vi "DAS.vi"() -> ()   [LabVIEW 2012]
uses:
  <vilib>/Utility/error.llb/DialogType.ctl
  SITK/Documents/SIToolkit/LabVIEW/Examples2012_4_1_0_4/Open-Close/CamHandle.vi
panel:
  in  "Record 3":bool
  in  "bUseBuffer1 3":bool
  in  "bUseBuffer0 3":bool
  in  "Record 2":bool
  in  "bUseBuffer1 2":bool
  in  "bUseBuffer0 2":bool
  in  "bUseBuffer0":bool
  in  "bUseBuffer1":bool
  in  "Open StructureIn":T1={"Size"=88, "InterfaceType"=0, "Camera Number"=0, "CameraNumAtInterface"=0, "OpenFlags"=[], "OpenDWFlags"=[], "OpenPtrs"=[]}
  out "Bits/pixel":u16
  out "BufNr1":i16
  out "BufNr0":i16
  in  "error in (no error)":errorcluster
  in  "Camera Handle 2":u32
  in  "File and Display Name 2":string
  in  "error in (no error) 2":errorcluster
  in  "Errors":errorcluster
  in  "?":T2(tab)
  out "Database Output":string
  out "Elapsed Time":u32
  in  "Image Tabs":T3(tab)
  out "Normalized Image":dbl[][](graph)
  out "Atoms":i16[][](graph)
  out "No Atoms":i16[][](graph)
  out "Dark Field":i16[][](graph)
  in  "?":T4(tab)
  in  "Cycle Devices (Red)\nAcquisition (Blue)":bool
  in  "?":bool
  in  "Scaling":dbl(slide)=0.0016108638057548662 scale=0.001..0.1
  in  "PF Scale":dbl(slide)=0.002000674655718671 scale=0.001..10.0
  in  "ADC Gain":i32=-1 min=-1 step=1
  in  "ADC Speed":i32=-1 min=-3 step=1
  in  "Exposure (sec)":dbl format="%.3f"
  in  "Number of Images":u32=1
  in  "Number of Accumulations":u32=1
  in  "Acquire / Focus Flag":u32(ring)=2 items=["Synchronous Focus Mode"=1, "Synchronous NFrame Mode"=2, "Asynchronous Mode"=3, "Sequence Mode"=4]
  in  "Timing Mode":u32(ring)=4 items=["Free Run"=1, "Trigger First"=2, "Strobe"=3, "Bulb"=4, "Variable"=5, "Flash"=6]
  in  "Trigger Edge":u32(ring)=1 items=["Rising"=1, "Falling"=2]
  in  "Milliseconds Between Shots":u32=200
  in  "InterfaceType":u16(ring)=6 items=["IEEE1394 - Firewire", "IEEE1394/Firewire", "Matrox Helios Camera Link", "Silicon Software ME3 Camera Link", "National Instruments Camera Link", "Gigabit Ethernet", "USB", "Reserved", "Reserved", "Reserved", "Generic Camera Link with CLSER.DLL"]
  in  "Rate":i32
  in  "ROIX1":u16=1 min=1
  in  "ROIY1":u16=1 min=1
  in  "ROIY0":u16=1 min=1
  in  "ROIX0":u16=1 min=1
  in  "DelayTimeBase":u16(ring)=2 items=["nanoseconds", "microseconds", "milliseconds"]
  in  "ExposureTimeBase":u16(ring)=1 items=["nanoseconds", "microseconds", "milliseconds"]
  in  "Exposure":u32=30
  in  "Delay":u32=100
  in  "StorageMode":bool
  in  "TriggerMode":u16(ring)=2 items=["Auto", "Software", "External sequence start ", "External exposure control"]
  out "Top of Chamber Monitor":dynamicdata(graph)
  in  "Image Tabs 2":T3(tab)
  out "Intensity Graph":dbl[][](graph)
  out "PF Atoms":u16[][](graph)
  out "PF No Atoms":u16[][](graph)
  out "PF Dark":u16[][](graph)
  # "Data Acquisition Suite v 1.3"
  # "Basic Output"
  # "Image Viewer"
  # "Image Viewer"
  # "DAS Mode Select"
  # "Stop Button"
  # "Experiment Setup"
  # "Advanced Setup"
  # "For everyday use, Number of Accumulations should be 1"
  # "Triggering Setup"
  # "Basic Setup for PixelFly"
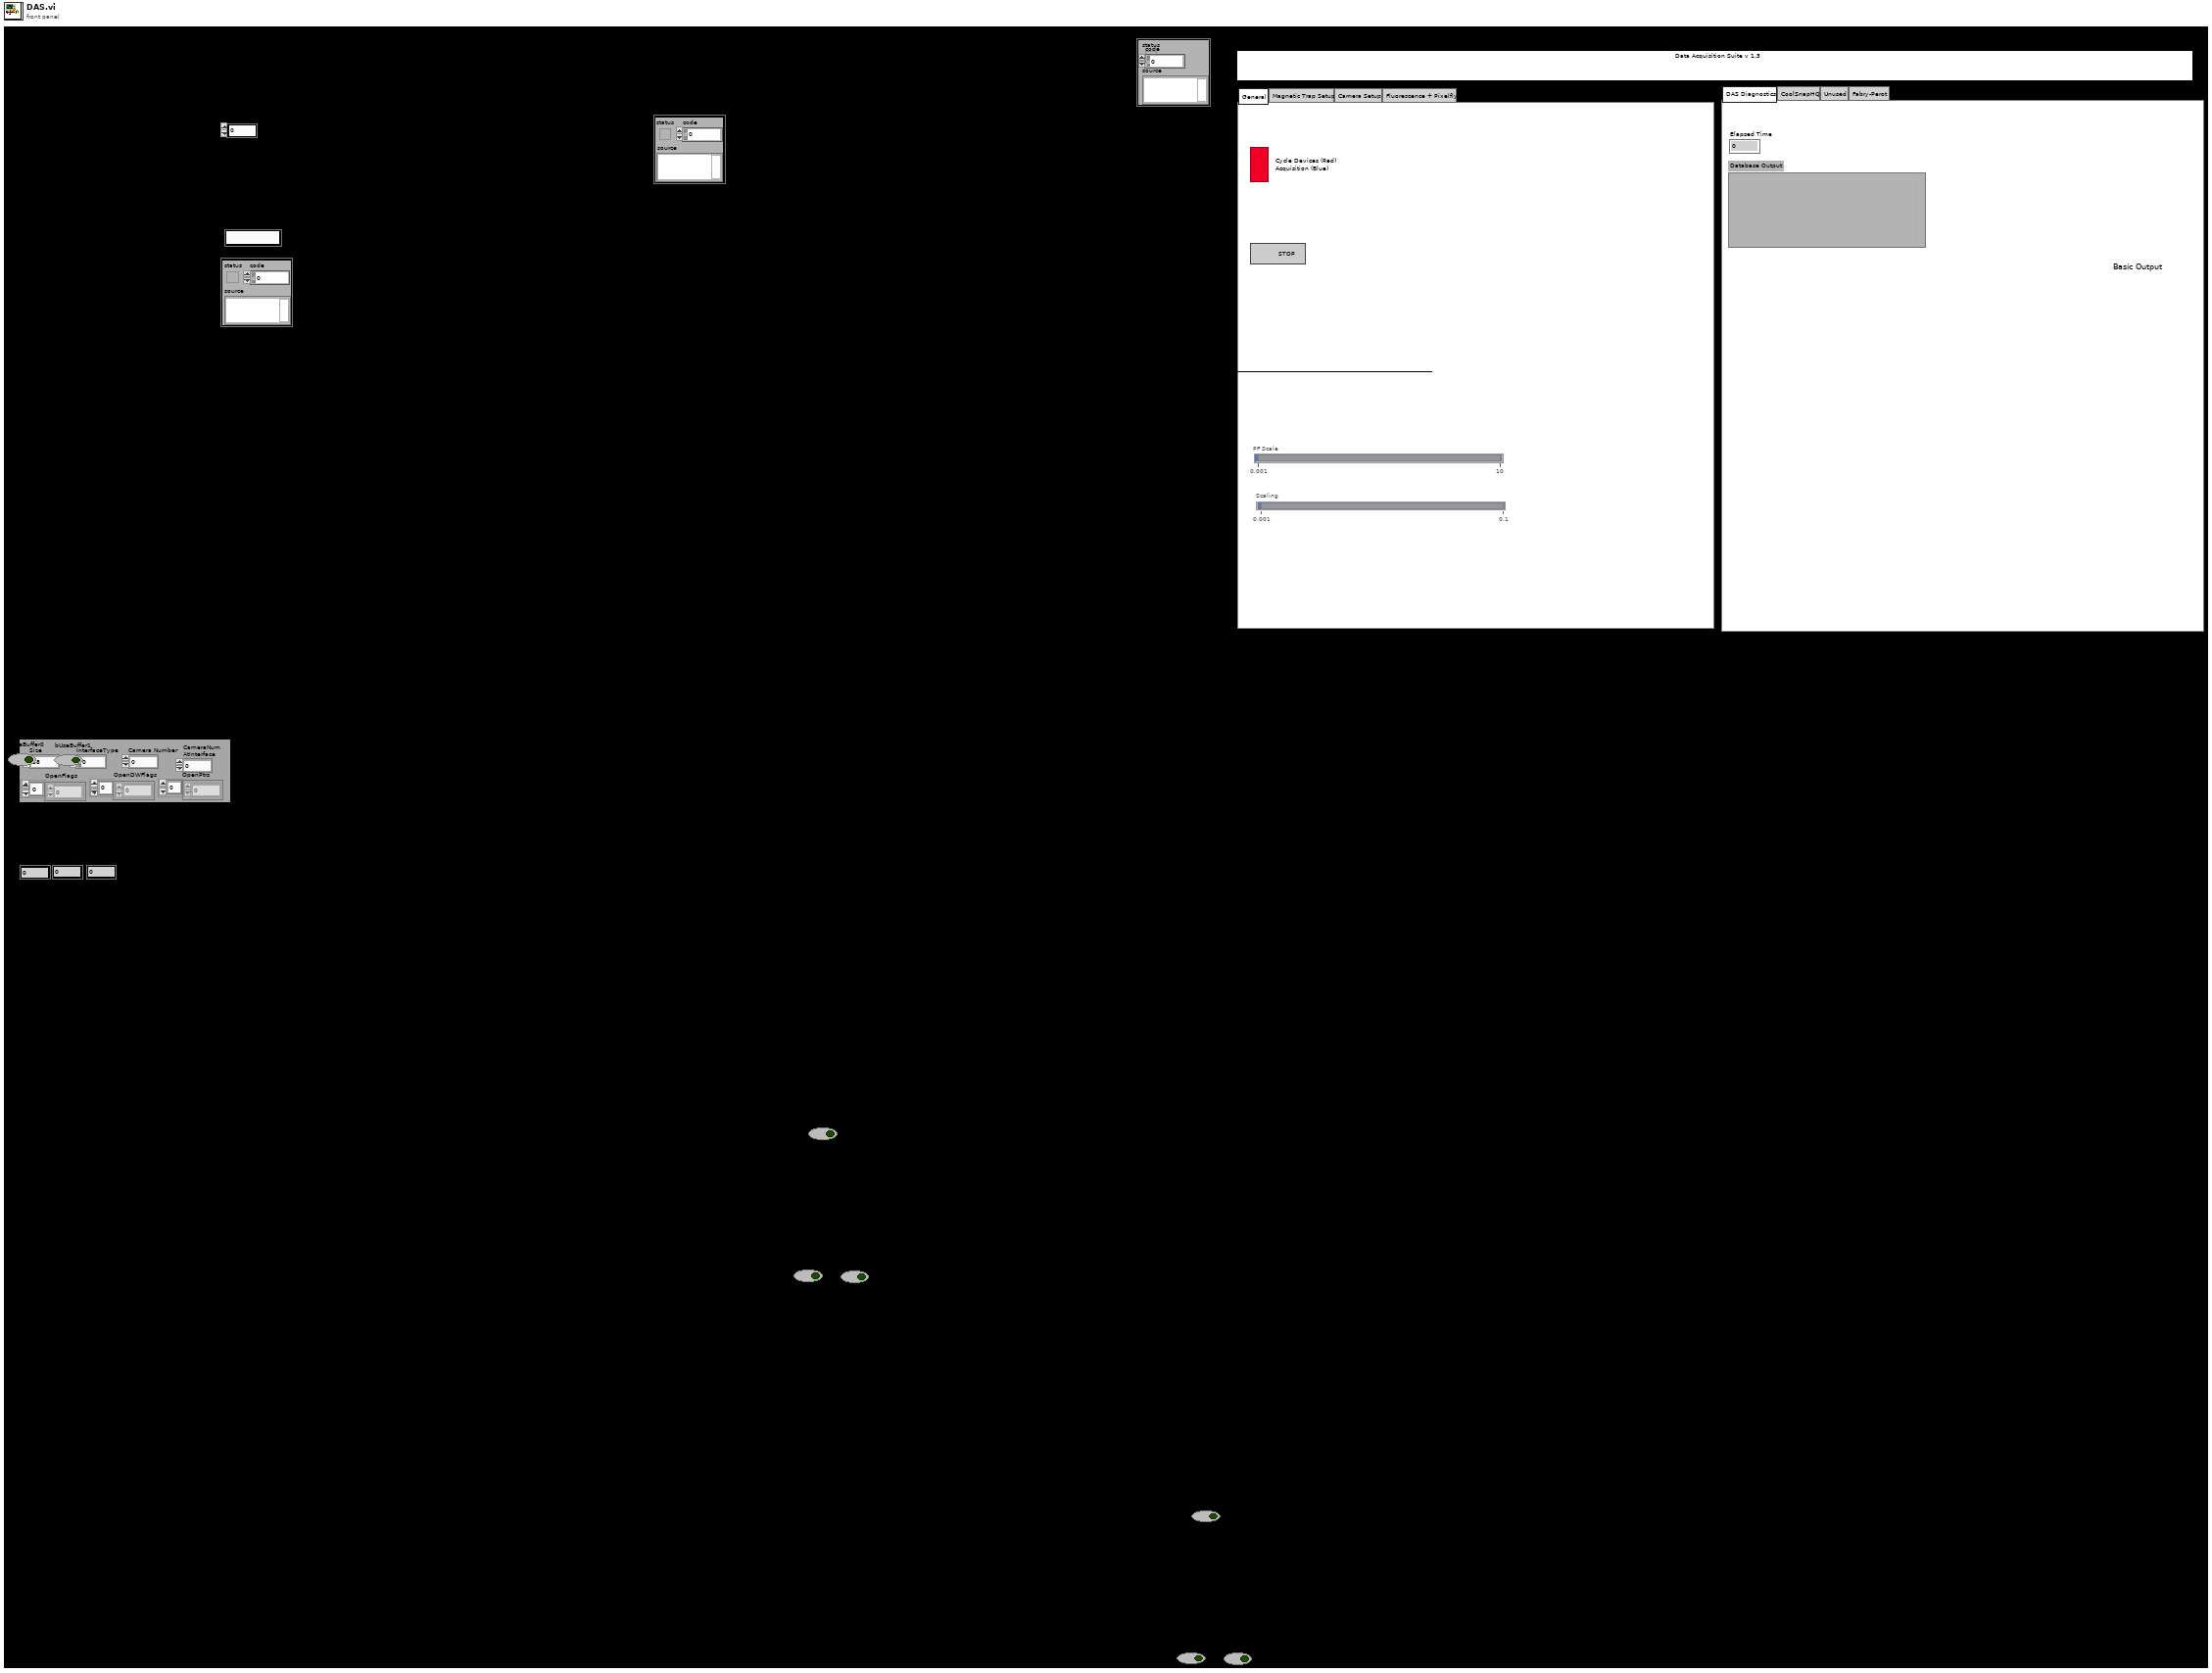
[diagram p1: front panel]
types:
  T1 = cluster{"Size":u16, "InterfaceType":u16, "Camera Number":u16, "CameraNumAtInterface":u16, "OpenFlags":u16[], "OpenDWFlags":u32[], "OpenPtrs":u32[]}
  T2 = enum32{"DAS Diagnostics", "CoolSnapHQ", "Unused", "Fabry-Perot"}
  T3 = enum32{"Composite Image", "Atoms", "No Atoms", "Dark Field"}
  T4 = enum32{"General", "Magnetic Trap Setup", "Camera Setup", "Fluorescence + Pixelfly"}
  T5 = enum16{"open", "replace", "create", "open or create", "replace or create", "replace or create with confirmation"}
  T6 = enum16{"big-endian, network order", "native, host order", "little-endian"}
  T7 = typedef "DialogType.ctl" = u16
  T8 = cluster{"Size":u16, "CamType":u16, "CamSubType":u16, "SerialNumber":u32, "HWVersion":u32, "FWVersion":u32, "InterfaceType":u16, "HardwareVersion":cluster{"BoardNum":u16, "HWVersions":cluster{"BoardName":string, "BatchNumber":u16, "MinorRevision":u8, "MajorRevision":u8, "Variant":u16}[]}, "FirmwareVersion":cluster{"DeviceNum":u16, "FWVersions":cluster{"DeviceName":string, "MinorRevision":u8, "MajorRevision":u8, "Variant":u16}[]}}
  T9 = cluster{"Size":u16, "SensorTypeDESC":u16, "SensorSubtypeDESC":u16, "MaxHorizontalResStdDESC":u16, "MaxVerticalResStdDESC":u16, "MaxHorizontalResExtDESC":u16, "MaxVerticalResExtDESC":u16, "DynResDESC":u16, "MaxBinHorzDESC":u16, "BinHorzStepDESC":bool, "MaxBinVertDESC":u16, "BinVertStepDESC":bool, "ROIHorzStepDESC":u16, "ROIVertStepDESC":u16, "NumADCDESC":u16, "IRDESC":bool, "MinDelayDESC":u32, "MaxDelayDESC":u32, "MinDelayStepDESC":u32, "MinExpoDESC":u32, "MaxExpoDESC":u32, "MinExpoStepDESC":u32, "MinDelayIRDESC":u32, "MaxDelayIRDESC":u32, "MinExpoIRDESC":u32, "MaxExpoIRDESC":u32, "TimeTableDESC":bool, "DoubleImageDESC":bool, "MinCoolSetDESC":i16, "MaxCoolSetDESC":i16, "MDefaultCoolSetDESC":i16, "PowerDownModeDESC":bool, "OffsetRegDESC":bool, "ColorPattern":cluster{"UpperLeftColor":u8, "UpperRightColor":u8, "LowerLeftColor":u8, "LowerRightColor":u8}, "PatternTypeDESC":bool, "PixelRates":u32[], "CoversionFactors":u16[], "Reserved":u32[], "NoiseFilterCapable":bool, "HotPixelCapable":bool, "HotPixelWithNoiseFilter":bool, "ASCIITimeCapable":bool, "Extended Description":bool, "Get Extended":bool, "Reserved Flag 1":bool, "Reserved Flag 2":bool}
  T10 = cluster{"Camera Handle":u32, "File Handle":u32, "Display Handle":u32, "Image Handle":u32}
  T11 = cluster{u16[][], "XResAct":u16, "YResAct":u16, "BufNrOut":i16, "BufNrOut":i16, "ErrorOut":errorcluster, "hout":u64, "Bits/pixel":u16}
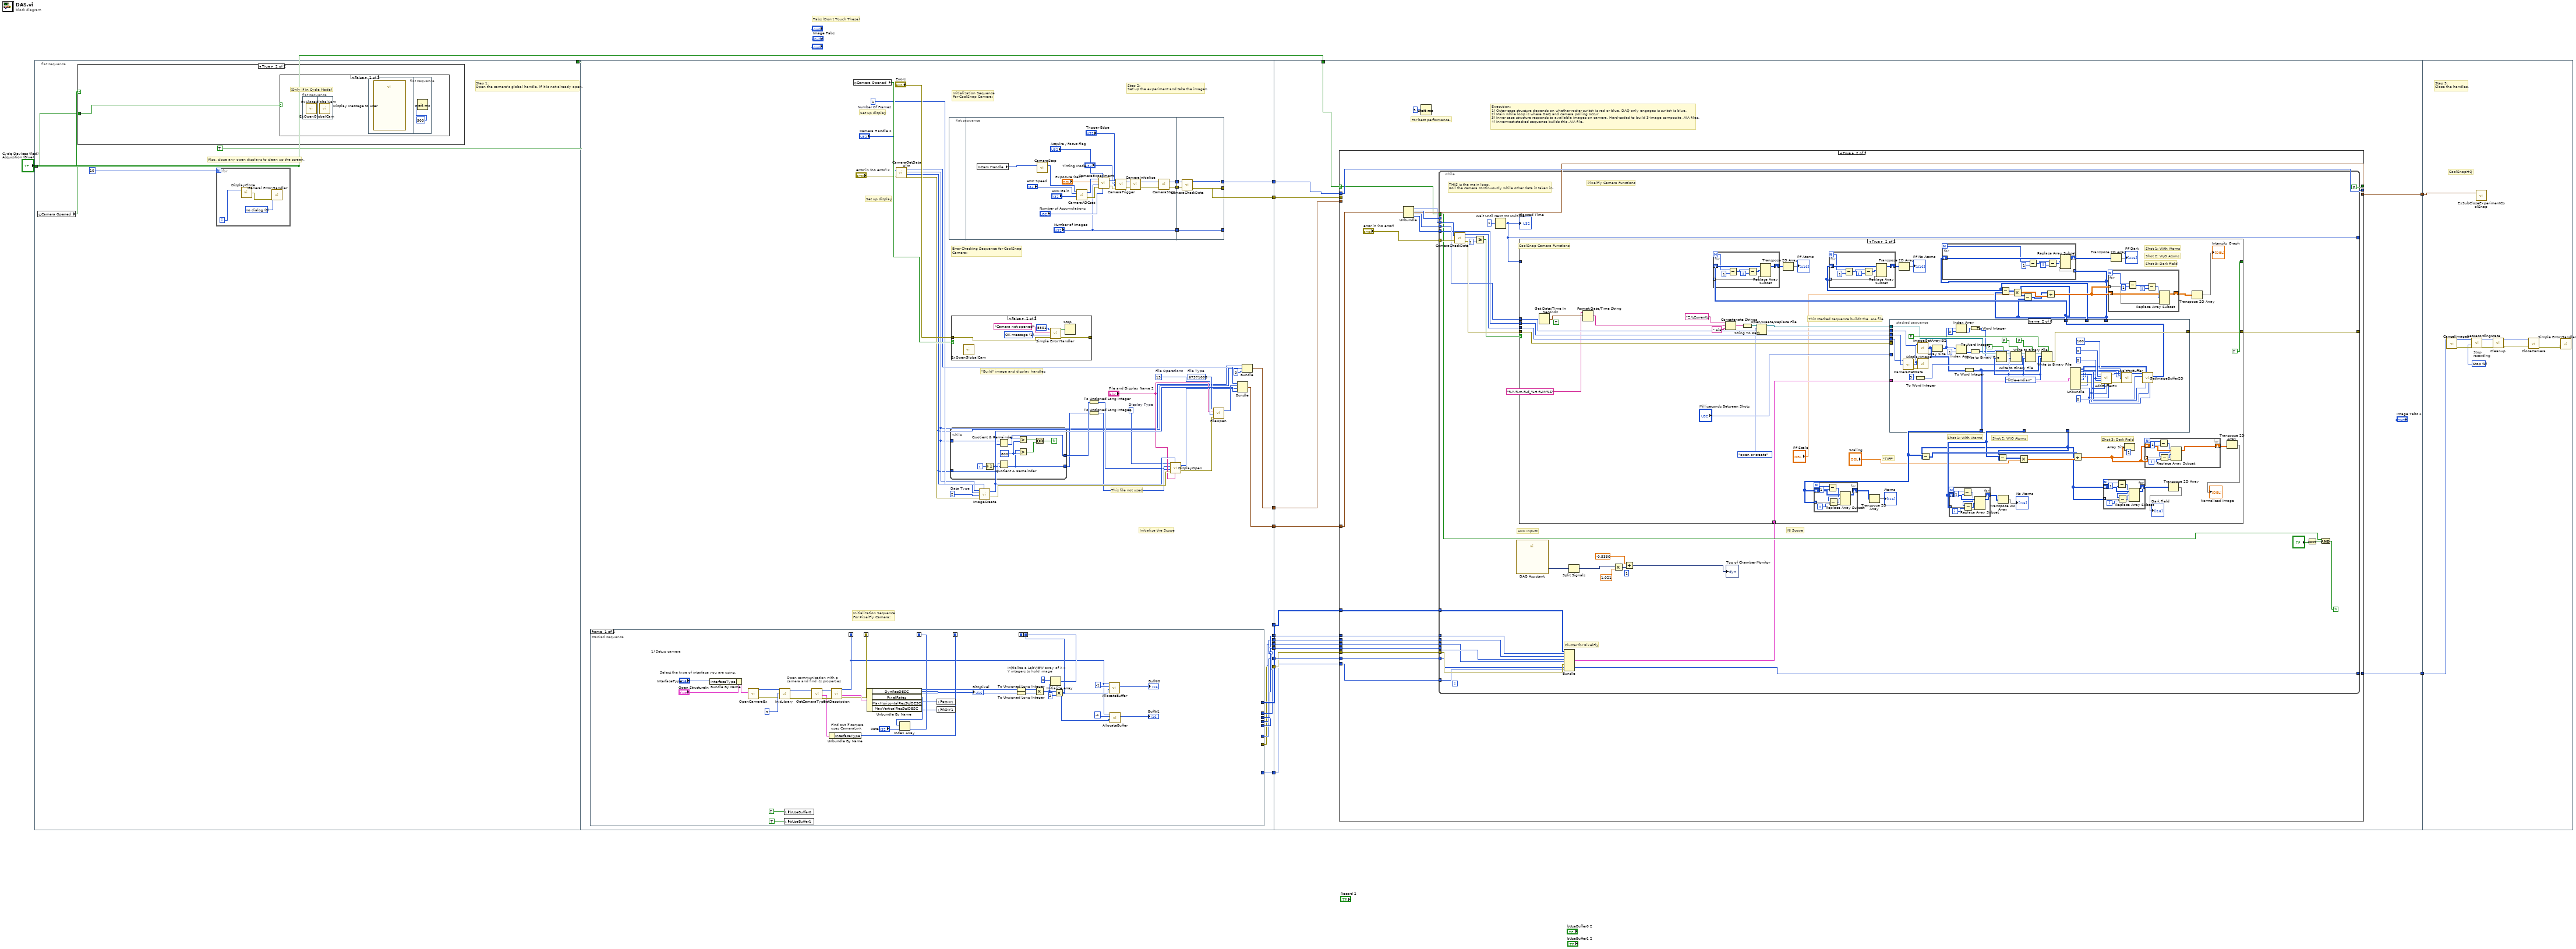
[diagram p0: block diagram]
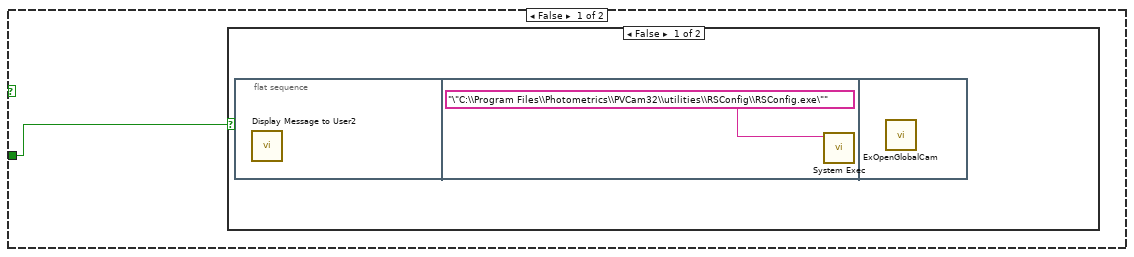
[diagram p2: hidden frame]
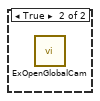
[diagram p3: hidden frame]
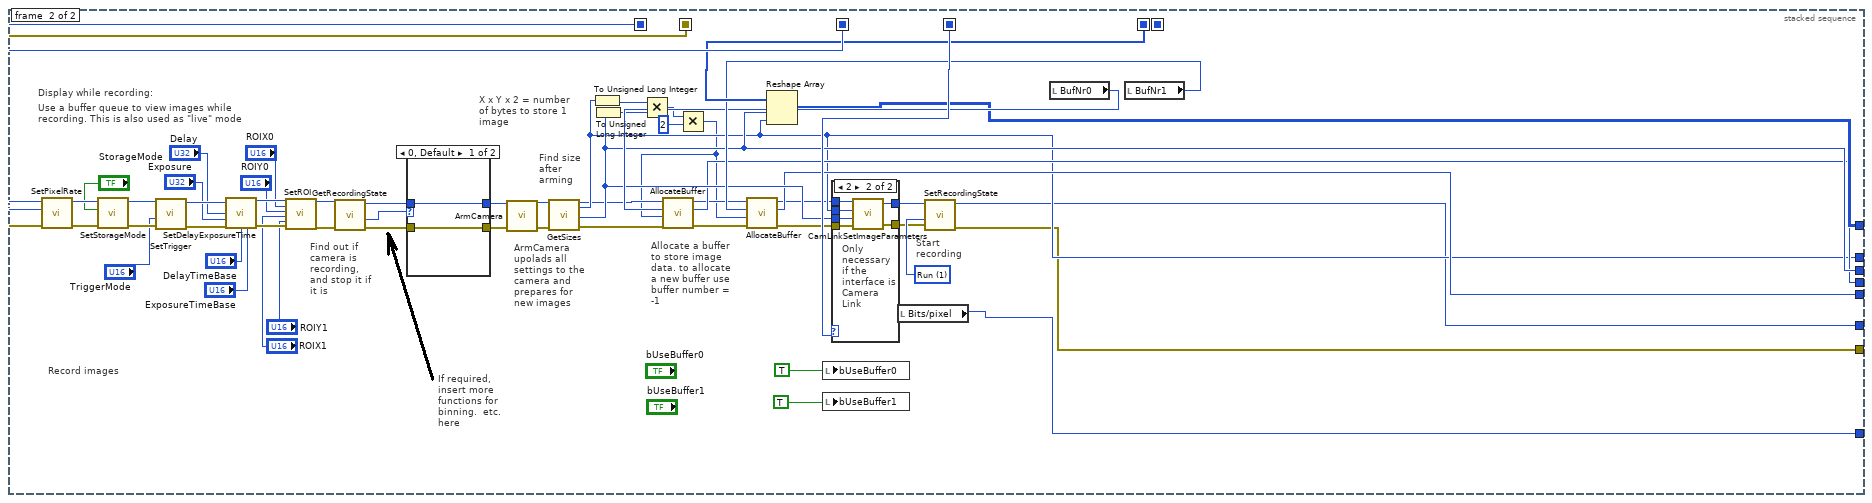
[diagram p5: hidden frame]
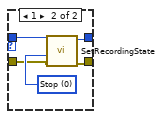
[diagram p7: hidden frame]
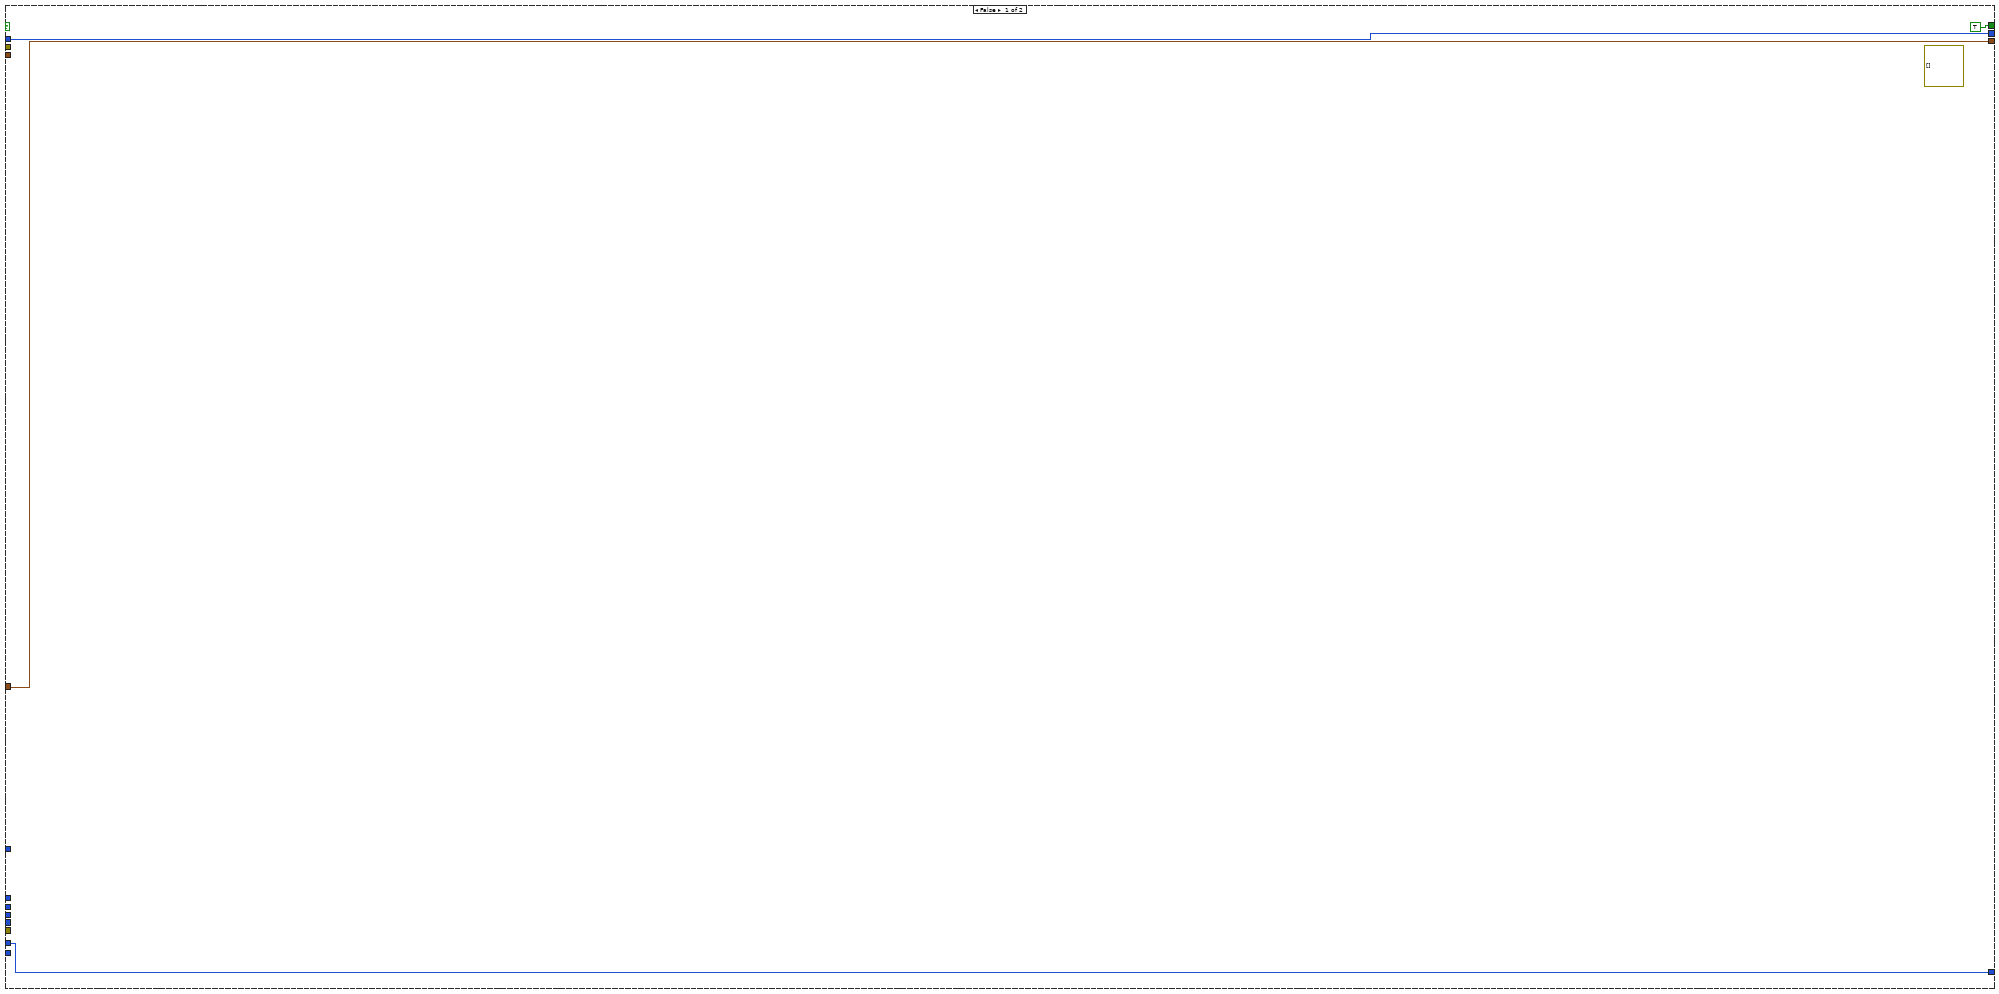
[diagram p9: hidden frame]
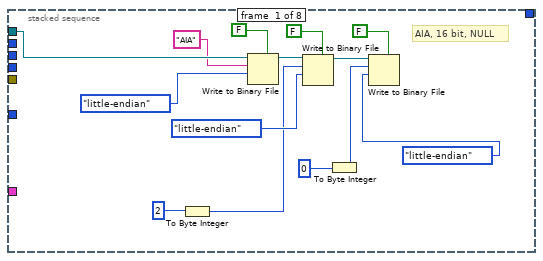
[diagram p11: hidden frame]
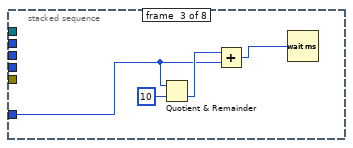
[diagram p12: hidden frame]
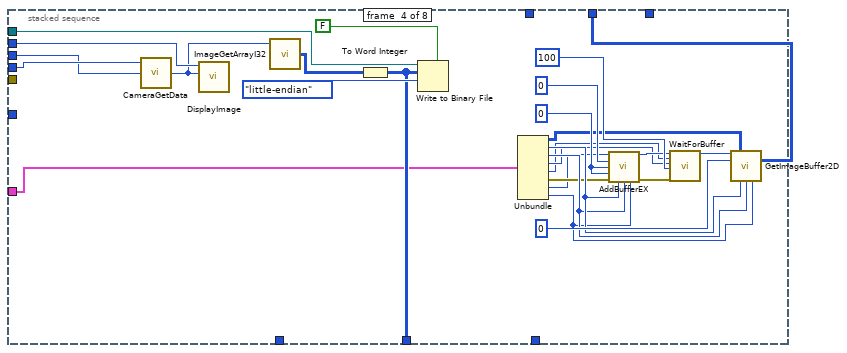
[diagram p13: hidden frame]
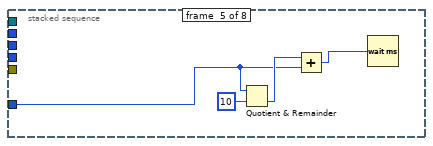
[diagram p14: hidden frame]
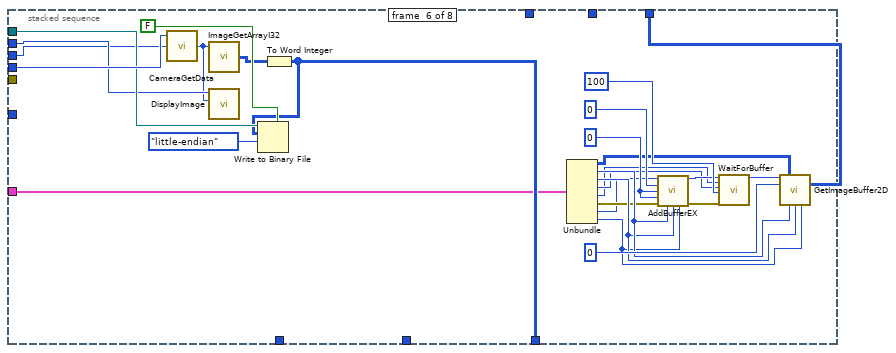
[diagram p15: hidden frame]
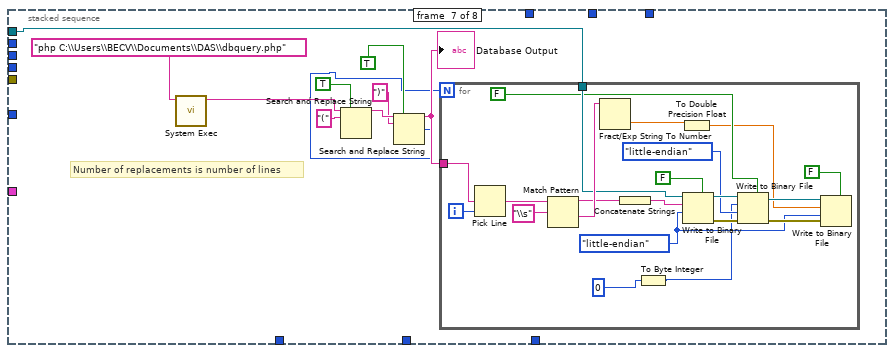
[diagram p16: hidden frame]
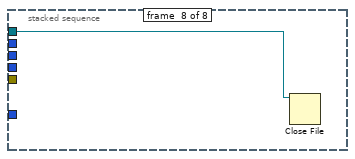
[diagram p17: hidden frame]
diagram:
  # "Tabs (Don't Touch These)"
  n1 = flat-sequence {
    tunnel: [TRUE] -> _
    tunnel: "Cycle Devices (Red)\nAcquisition (Blue)" -> [w16]
    tunnel: [w39] -> w15
    tunnel: [w38] -> w14
    tunnel: [w37] -> w13
    tunnel: [w36] -> w12
    tunnel: [w35] -> w9
    tunnel: [w34] -> w8
    tunnel: [w33] -> w7
    tunnel: [w32] -> w6
    tunnel: [w31] -> w5
    tunnel: [w30] -> w4
    tunnel: [w29] -> w3
    tunnel: [w28] -> w2
    tunnel: w15 -> [w230]
    tunnel: w14 -> [w226]
    tunnel: w13 -> [w229]
    tunnel: w12 -> [w228]
    tunnel: [w227] -> w11
    tunnel: "Cycle Devices (Red)\nAcquisition (Blue)" -> [w224]
    tunnel: w9 -> [w223]
    tunnel: w8 -> [w222]
    tunnel: w7 -> [w221]
    tunnel: w6 -> [w220]
    tunnel: w5 -> [w219]
    tunnel: w4 -> [w218]
    tunnel: w3 -> [w217]
    tunnel: w2 -> [w216]
    tunnel: [w215] -> w1
    tunnel: w11 -> [w557]
    tunnel: w1 -> [w553]
    frame #0 {
      # "Also, close any open displays to clean up the screen."
      # "Step 1:\nOpen the camera's global handle, if it is not already open."
      n2 = global read "CamHandle.vi" "Camera Opened"() -> (w19:bool)
      n3 = case shown="True" w19 {
        tunnel: w16 -> [w23 w25]
        frame False {
          n4 = case shown="False" w23 {
            frame False {
              n5 = flat-sequence {
                frame #0 {
                  n6 = call "Display Message to User2"() -> ()  [unwired: 10 in, 2 out]
                }
                frame #1 {
                  n7 = call <vilib>:"System Exec.vi"("command line"="\"C:\\Program Files\\Photometrics\\PVCam32\\utilities\\RSConfig\\RSConfig.exe\"") -> ()  [unwired: 7 in, 4 out]
                }
                frame #2 {
                  n8 = call "ExOpenGlobalCam.vi"() -> ()  [unwired: 1 in]
                }
              }
            }
            frame True {
              n9 = call "ExOpenGlobalCam.vi"() -> ()  [unwired: 1 in]
            }
          }
        }
        frame True {
          n10 = case shown="False" w25 {
            frame False {
              # "(Only if in Cycle Mode)"
              n11 = flat-sequence {
                frame #0 {
                  n12 = call "ExCloseGlobalCam.vi"() -> ()  [unwired: 1 in]
                }
                frame #1 {
                  n13 = call "ExOpenGlobalCam.vi"() -> ()  [unwired: 1 in]
                }
              }
              n14 = flat-sequence {
                frame #0 {
                  n15 = call "Display Message to User"() -> ()  [unwired: 10 in, 2 out]
                }
                frame #1 {
                  n16 = Wait (ms)(milliseconds to wait=u32 500) -> ()  [unwired: 1 out]
                }
              }
            }
            frame True {
            }
          }
        }
      }
      n17 = for {
        N: 10 -> [_]
        i -> [w22]
        w20 = T7 0 items=["no dialog", "OK message", "continue or stop message", "OK message + warnings", "continue/stop + warnings"] ("type of dialog (OK msg:1)")
        n18 = call <userlib>:"DisplayClose.vi"("Display Handle"=w22) -> ("error out"=w21:errorcluster)  [unwired: 1 in]
        n19 = call <vilib>:"General Error Handler.vi"("type of dialog (OK msg:1)"=w20, "error in (no error)"=w21) -> ()  [unwired: 9 in, 5 out]
      }
    }
    frame #1 {
      w50 = u32 1  # Number Of Frames
      w51 = u32 4  # Display Type
      w52 = u32 2  # Data Type
      w54 = 13  # File Operations
      w55 = 67371008  # File Type
      # "Initialization Sequence \nFor PixelFly Camera:"
      # "Initialize the Scope"
      # "Error Checking Sequence for CoolSnap\nCamera:"
      # "Initialization Sequence \nFor CoolSnap Camera:"
      # "This file not used"
      # "\"Build\" image and display handles"
      # "Set up display"
      # "Set up display"
      # "Step 2:\nSet up the experiment and take the images."
      n20 = stacked-sequence {
        seq-local: [w96 _] -> [_ w154]
        seq-local: [w77 _] -> [_ _]
        seq-local: [w89 _] -> [_ w156]
        seq-local: [w76 _] -> [_ w151]
        seq-local: [w88 _] -> [_ w157]
        seq-local: [w87 _] -> [_ w155]
        tunnel: [_ w150] -> w35
        tunnel: [_ w146] -> w34
        tunnel: [_ w149] -> w33
        tunnel: [_ w148] -> w32
        tunnel: [_ w147] -> w31
        tunnel: [_ w145] -> w30
        tunnel: [_ w144] -> w29
        tunnel: [_ w143] -> w28
        frame #0 {
          # "Select the type of interface you are using."
          # "1) Setup camera"
          # "Find out if camera uses CameraLink"
          # "Initialize a LabVIEW array of X x Y integers to hold image"
          # "Open communication with a camera and find its properties"
          n21 = Bundle By Name(cluster="Open StructureIn", "InterfaceType"="InterfaceType") -> (w84:T1)
          n22 = call "OpenCameraEx.vi"("OpenStructureIn"=w84) -> ("error out"=w68:errorcluster, "hout"=w69:u64)  [unwired: 3 in, 2 out]
          n23 = call "InitLibrary.vi"("error in (no error)"=w68, "InterfaceType"=u32 3, "ph"=w69) -> ("error out"=w66:errorcluster, "hout"=w67:u64)  [unwired: 7 in]
          n24 = local write "bUseBuffer0"(TRUE) -> ()
          n25 = local write "bUseBuffer1"(TRUE) -> ()
          n26 = call "GetCameraType.vi"("ph"=w67, "error in (no error)"=w66) -> ("hout"=w93:u64, "CameraType"=w91:T8, "error out"=w92:errorcluster)  [unwired: 1 in, 1 out]
          n27 = Unbundle By Name(w91) -> ("InterfaceType"=w87:u16)
          n28 = call "GetDescription.vi"("ErrorIn"=w92, "ph"=w93) -> ("ErrorOut"=w88:errorcluster, "Description"=w95:T9, "hout"=w76:u64)  [unwired: 2 in, 1 out]
          n29 = Unbundle By Name(w95) -> ("DynResDESC"=→"Bits/pixel":u16, "PixelRates"=w90:u32[], "MaxHorizontalResStdDESC"=w82:u16, "MaxVerticalResStdDESC"=w81:u16)
          n30 = Index Array(array=w90, index="Rate") -> (element=w89:u32)
          n31 = local write "ROIX1"(w82) -> ()
          n32 = local write "ROIY1"(w81) -> ()
          n33 = To Unsigned Long Integer(number=w82) -> (unsigned 32bit integer=w79:u32)
          n34 = To Unsigned Long Integer(number=w81) -> (unsigned 32bit integer=w78:u32)
          n35 = Multiply(x=w79, y=w78) -> (x*y=w97:u32)
          n36 = Initialize Array(u16 0 ("Element Data"), w97) -> (w96:u16[])
          n37 = Multiply(x=w97, y=u32 2) -> (x*y=w77:u32)
          n38 = call "AllocateBuffer.vi"("Size"=w77, "BufNr"=i16 -1, "ph"=w76) -> ("BufNrOut"=→"BufNr0":i16)  [unwired: 3 in, 5 out]
          n39 = call "AllocateBuffer.vi"("Size"=w77, "BufNr"=-1, "ph"=w76) -> ("BufNrOut"=→"BufNr1":i16)  [unwired: 3 in, 5 out]
        }
        frame #1 {
          w142 = u16 1 items=["Stop", "Run"] ("RecordingState")
          # "Record images"
          # "Start recording"
          # "Allocate a buffer to store image data. to allocate a new buffer use buffer number = -1"
          # "Find size after arming"
          # "ArmCamera upolads all settings to the camera and prepares for new images"
          # "Find out if camera is recording, and stop it if it is"
          # "If required, insert more functions for binning.  etc. here"
          # "X x Y x 2 = number of bytes to store 1 image"
          # "Use a buffer queue to view images while recording. This is also used as \"live\" mode"
          # "Display while recording:"
          n40 = call "SetPixelRate.vi"("error in (no error)"=w157, "PixelRate"=w156, "ph"=w151) -> ("error out"=w140:errorcluster, "hout"=w141:u64)  [unwired: 2 in, 1 out]
          n41 = call "SetStorageMode.vi"("error in (no error)"=w140, "StorageMode"="StorageMode", "ph"=w141) -> ("error out"=w132:errorcluster, "hout"=w133:u64)  [unwired: 2 in, 1 out]
          n42 = call "SetTrigger.vi"("error in (no error)"=w132, "TriggerMode"="TriggerMode", "ph"=w133) -> ("error out"=w125:errorcluster, "hout"=w126:u64)  [unwired: 2 in, 1 out]
          n43 = call "SetDelayExposureTime.vi"("ph"=w126, "Delay"="Delay", "Exposure"="Exposure", "error in (no error)"=w125, "DelayTimeBase"="DelayTimeBase", "ExposureTimeBase"="ExposureTimeBase") -> ("hout"=w114:u64, "error out"=w112:errorcluster)  [unwired: 7 in, 1 out]
          n44 = call "SetROI.vi"("ph"=w114, "ROIX0"="ROIX0", "ROIY0"="ROIY0", "ROIX1"="ROIX1", "ROIY1"="ROIY1", "error in (no error)"=w112) -> ("hout"=w113:u64, "error out"=w111:errorcluster)  [unwired: 12 in]
          n45 = call "GetRecordingState.vi"("ErrorIn"=w111, "ph"=w113) -> ("ErrorOut"=w136:errorcluster, "RecordingState"=w138:u16, "hout"=w137:u64)  [unwired: 2 in, 1 out]
          n46 = case shown="0, Default" w138 {
            tunnel: w137 -> [w167 w171]
            tunnel: w136 -> [w166 w170]
            tunnel: [w167 w169] -> w135
            tunnel: [w166 w168] -> w134
            frame 0, Default {
            }
            frame 1 {
              w172 = u16 0 items=["Stop", "Run"] ("RecordingState")
              n47 = call "SetRecordingState.vi"("ErrorIn"=w170, "RecordingState"=w172, "ph"=w171) -> ("ErrorOut"=w168:errorcluster, "hout"=w169:u64)  [unwired: 2 in, 1 out]
            }
          }
          n48 = call "ArmCamera.vi"("error in (no error)"=w134, "ph"=w135) -> ("error out"=w130:errorcluster, "hout"=w131:u64)  [unwired: 1 in, 1 out]
          n49 = call "GetSizes.vi"("ph"=w131, "ErrorIn"=w130) -> ("hout"=w127:u64, "XResAct"=w146:u16, "YResAct"=w149:u16, "ErrorOut"=w129:errorcluster)  [unwired: 11 in, 3 out]
          n50 = To Unsigned Long Integer(number=w146) -> (unsigned 32bit integer=w115:u32)
          n51 = To Unsigned Long Integer(number=w149) -> (unsigned 32bit integer=w116:u32)
          n52 = Multiply(x=w115, y=w116) -> (x*y=w117:u32)
          n53 = Multiply(x=w117, y=u32 2) -> (x*y=w102:u32)
          n54 = Reshape Array(w154, w149, w146) -> (w150:u16[][])
          n55 = local write "bUseBuffer0"(TRUE) -> ()
          n56 = local write "bUseBuffer1"(TRUE) -> ()
          n57 = local read "Bits/pixel"() -> (w143:u16)
          n58 = local read "BufNr0"() -> (w152:i16)
          n59 = call "AllocateBuffer.vi"("error in (no error)"=w129, "Size"=w102, "BufNr"=w152, "ph"=w127) -> ("error out"=w106:errorcluster, "BufNrOut"=w148:i16, "hout"=w104:u64)  [unwired: 2 in, 3 out]
          n60 = local read "BufNr1"() -> (w153:i16)
          n61 = call "AllocateBuffer.vi"("error in (no error)"=w106, "Size"=w102, "BufNr"=w153, "ph"=w104) -> ("error out"=w105:errorcluster, "BufNrOut"=w147:i16, "hout"=w103:u64)  [unwired: 2 in, 3 out]
          n62 = case shown="2" w155 {
            tunnel: w105 -> [w158 w165]
            tunnel: [w158 w164] -> w120
            tunnel: w103 -> [w159 w163]
            tunnel: [w159 w162] -> w119
            tunnel: w149 -> [_ w161]
            tunnel: w146 -> [_ w160]
            frame 0, Default {
            }
            frame 2 {
              # "Only necessary if the interface is Camera Link"
              n63 = call "CamLinkSetImageParameters.vi"("error in (no error)"=w165, "YRes"=w161, "XRes"=w160, "ph"=w163) -> ("error out"=w164:errorcluster, "hout"=w162:u64)  [unwired: 1 out]
            }
          }
          n64 = call "SetRecordingState.vi"("ErrorIn"=w120, "RecordingState"=w142, "ph"=w119) -> ("ErrorOut"=w144:errorcluster, "hout"=w145:u64)  [unwired: 2 in, 1 out]
        }
      }
      n65 = global read "CamHandle.vi" "Camera Opened"() -> (w65:bool)
      n66 = call <userlib>:"CameraGetDataDim.vi"("Camera Handle"="Camera Handle 2", "error in"="error in (no error) 2") -> ("Camera Handle"=w58:u32, "Xdim"=w42:u32, "Ydim"=w41:u32, "error out"=w63:errorcluster)
      n67 = flat-sequence {
        tunnel: ["Number of Images"] -> w45
        tunnel: [w179] -> w44
        tunnel: [w178] -> w43
        tunnel: [w193] -> w37
        tunnel: [w197] -> _
        tunnel: w45 -> [w197]
        tunnel: w44 -> [w196]
        tunnel: w43 -> [w195]
        tunnel: [w194] -> w36
        frame #0 {
        }
        frame #1 {
          n68 = global read "CamHandle.vi" "Cam Handle"() -> (w173:u32)
          n69 = call <userlib>:"CameraStop.vi"("Camera Handle"=w173) -> ("Camera Handle"=w174:u32)  [unwired: 1 in, 1 out]
          n70 = call <userlib>:"CameraADCset.vi"("ADC Gain"="ADC Gain", "ADC Speed"="ADC Speed", "Camera Handle"=w174) -> ("error out"=w190:errorcluster, "Camera Handle"=w192:u32)  [unwired: 3 in]
          n71 = call <userlib>:"CameraExperiment.vi"("Number of Accumulations"="Number of Accumulations", "Acquire / Focus Flag"="Acquire / Focus Flag", "error in"=w190, "Number of Images"="Number of Images", "Exposure (sec)"="Exposure (sec)", "Camera Handle"=w192) -> ("error out"=w184:errorcluster, "Camera Handle"=w185:u32)
          n72 = call <userlib>:"CameraTrigger.vi"("error in"=w184, "Trigger Edge"="Trigger Edge", "Timing Mode"="Timing Mode", "Camera Handle"=w185) -> ("error out"=w175:errorcluster, "Camera Handle"=w180:u32)
          n73 = call <userlib>:"CameraInitialize.vi"("error in"=w175, "Camera Handle"=w180) -> ("error out"=w177:errorcluster, "Camera Handle"=w176:u32)
          n74 = call <userlib>:"CameraStart.vi"("error in"=w177, "Camera Handle"=w176) -> ("error out"=w178:errorcluster, "Camera Handle"=w179:u32)
        }
        frame #2 {
          n75 = call <userlib>:"CameraCheckData.vi"("Camera Handle"=w196, "error in"=w195) -> ("Camera Handle"=w193:u32, "error out"=w194:errorcluster)  [unwired: 1 out]
        }
      }
      n76 = while {
        tunnel: w42 -> [w206]
        tunnel: w41 -> [w205]
        tunnel: [w200] -> w49
        tunnel: [w199] -> w48
        i -> [w204]
        stop <- w201 continue-if-true
        w207 = 800
        n77 = Increment(x=w204) -> (x+1=w198:i32)
        n78 = Quotient & Remainder(x=w206, y=w198) -> (floor(x/y)=w200:u32)  [unwired: 1 out]
        n79 = Quotient & Remainder(x=w205, y=w198) -> (floor(x/y)=w199:u32)  [unwired: 1 out]
        n80 = Greater?(x=w200, y=w207) -> (0:w203:bool)
        n81 = Greater?(x=w199, y=w207) -> (0:w202:bool)
        n82 = Or(x=w203, y=w202) -> (x .or. y?=w201:bool)
      }
      n83 = case shown="False" w65 {
        tunnel: [w212 w214] -> _
        tunnel: "Errors" -> [w208 w214]
        frame False {
          w213 = u16 1 items=["no dialog", "OK message", "continue or stop message"] ("type of dialog (OK msg:1)")
          n84 = call "ExOpenGlobalCam.vi"() -> ()  [unwired: 1 in]
          n85 = call <vilib>:"Simple Error Handler.vi"("error code (no error:0)"=5501, "error source (\" \")"="Camera not opened", "type of dialog (OK msg:1)"=w213, "error in (no error)"=w208) -> ("error?"=w210:bool, "error out"=w212:errorcluster)  [unwired: 1 in, 3 out]
          n86 = Stop(stop? (T)=w210) -> ()
        }
        frame True {
        }
      }
      n87 = call <userlib>:"ImageCreate.vi"("X dimension"=w42, "Y dimension"=w41, "Data Type"=w52, "error in"=w63, "Number Of Frames"=w50) -> ("Image Handle"=w56:u32, "error out"=w62:errorcluster)
      n88 = To Unsigned Long Integer(number=w49) -> (unsigned 32bit integer=w47:u32)
      n89 = To Unsigned Long Integer(number=w48) -> (unsigned 32bit integer=w46:u32)
      n90 = call <userlib>:"DisplayOpen.vi"("Display Title"="File and Display Name 2", "Image Handle"=w56, "error in"=w62, "Display Height"=w46, "Display Width"=w47, "Display Type"=w51) -> ("error out"=w61:errorcluster, "Display Handle"=w27:u32)
      n91 = call <userlib>:"FileOpen.vi"("error in"=w61, "File Operations"=w54, "FileName"="File and Display Name 2", "File Type"=w55) -> ("File Handle"=w57:u32)  [unwired: 1 out]
      n92 = Bundle("Camera Handle"=w58, "File Handle"=w57, "Display Handle"=w27, "Image Handle"=w56) -> (w38:T10)  [unwired: 1 in]
      n93 = Bundle("Xdim"=w42, "Ydim"=w41, 0) -> (w39:cluster{"Xdim":u32, "Ydim":u32, i32})  [unwired: 1 in]
    }
    frame #2 {
      # "For best performance."
      # "Execution:\n1) Outer case structure depends on whether rocker switch is red or blue. DAQ only engages is switch is blue.\n2) Main while loop is where DAQ and camera polling occur\n3) Inner case structure responds to available images on camera. Hard-coded to build 3-image composite .AIA files.\n4) Innermost stacked sequence builds this .AIA file."
      n94 = case shown="True" w224 {
        selector: w224 -> [_ w244]
        tunnel: w226 -> [w234 w246]
        tunnel: [w234 w246] -> w227
        tunnel: w229 -> [w233 w251]
        tunnel: w228 -> [_ _]
        tunnel: [w233 w251] -> _
        tunnel: [TRUE FALSE] -> _
        tunnel: w230 -> [_ _]
        tunnel: w223 -> [_ w243]
        tunnel: w222 -> [_ w242]
        tunnel: w221 -> [_ w241]
        tunnel: w220 -> [_ w240]
        tunnel: w219 -> [_ w239]
        tunnel: w218 -> [w231 w238]
        tunnel: w217 -> [_ w237]
        tunnel: w216 -> [_ w236]
        tunnel: [w231 w235] -> w215
        frame False {
          (unwired) errorcluster[] []
        }
        frame True {
          n95 = Unbundle(w246) -> ("Camera Handle"=w245:u32, "File Handle"=w249:u32, "Display Handle"=w248:u32, "Image Handle"=w247:u32)
          n96 = while {
            tunnel: "error in (no error)" -> [w283]
            tunnel: w245 -> [w282]
            tunnel: [w279] -> _
            tunnel: w249 -> [_]
            tunnel: w248 -> [w278]
            tunnel: w247 -> [w277]
            tunnel: [w275] -> _
            tunnel: w244 -> [w265]
            tunnel: w243 -> [w261]
            tunnel: w242 -> [w260]
            tunnel: w241 -> [w259]
            tunnel: w240 -> [w257]
            tunnel: w239 -> [w258]
            tunnel: w238 -> [w253]
            tunnel: w237 -> [w256]
            tunnel: w236 -> [w255]
            tunnel: [w253] -> w235
            stop <- w264 continue-if-true
            (unwired) 1
            # "Cluster for PixelFly"
            # "PixelFly Camera Functions"
            # "NI Scope"
            # "CoolSnap Camera Functions"
            # "ADC Inputs"
            # "THIS is the main loop.\nPoll the camera continuously while other data is taken in."
            n97 = call <userlib>:"CameraCheckData.vi"("Camera Handle"=w282, "error in"=w283) -> ("Camera Handle"=w281:u32, "Number Of Frames Available"=w274:i32, "error out"=w280:errorcluster)
            n98 = Greater Or Equal?(x=w274, y=1) -> (x >= y?=w272:bool)
            n99 = Wait Until Next ms Multiple(millisecond multiple=1) -> (millisecond timer value=w275:u32)
            "Elapsed Time" <- w275
            n100 = call "DAQ Assistant"() -> ("data"=w271:dynamicdata)  [unwired: 17 in, 2 out]
            n101 = Bundle(w261, "XResAct"=w260, "YResAct"=w259, "BufNrOut"=w258, "BufNrOut"=w257, "ErrorOut"=w256, "hout"=w253, "Bits/pixel"=w255) -> (w254:T11)  [unwired: 1 in]
            n102 = case shown="True" w272 {
              selector: w272 -> [w284 _]
              tunnel: w281 -> [_ w334]
              tunnel: w280 -> [w285 w333]
              tunnel: [w284 TRUE] -> _
              tunnel: [w285 w323] -> w279
              tunnel: w278 -> [_ w332]
              tunnel: w277 -> [_ w329]
              tunnel: w275 -> [_ _]
              tunnel: w254 -> [_ w313]
              frame False {
              }
              frame True {
                (unwired) 1 ("index")
                (unwired) TRUE ("want seconds? (F)")
                # "Shot 1: With Atoms"
                # "Shot 3: Dark Field"
                # "Shot 2: W/O Atoms"
                # "Shot 3: Dark Field"
                # "Shot 2: W/O Atoms"
                # "Shot 1: With Atoms"
                # "This stacked sequence builds the .AIA file"
                # "\"TIFF\""
                n103 = Get Date/Time In Seconds() -> (seconds since 1Jan1904=w316:timestamp)
                n104 = Format Date/Time String(time format string (%c)="%Y-%m-%d_%H;%M;%S", seconds (now)=w316) -> (date/time string=w314:string)  [unwired: 1 in]
                n105 = Concatenate Strings("Z:\\Current\\" ("string"), w314, ".aia" ("string")) -> (w327:string)
                n106 = String To Path(string=w327) -> (path=w326:path)
                n107 = Open/Create/Replace File(file path (use dialog)=w326, operation (0:open)=T5."open or create") -> (refnum out=w325:refnum<file>)  [unwired: 4 in, 2 out]
                n108 = stacked-sequence {
                  tunnel: w334 -> [_ w452 _ w485 _ w515 _ _]
                  tunnel: w333 -> [_ _ _ _ _ _ _ _]
                  tunnel: w332 -> [_ w454 _ w482 _ w512 _ _]
                  tunnel: w329 -> [_ w453 _ w481 _ w511 _ _]
                  tunnel: w325 -> [w412 w446 _ w483 _ w513 w517 w547]
                  tunnel: [_ w449 _ _ _ _ _ _] -> w323
                  tunnel: "Milliseconds Between Shots" -> [_ _ w456 _ w486 _ _ _]
                  tunnel: [_ w430 _ _ _ _ _ _] -> w309
                  tunnel: [_ _ _ w477 _ _ _ _] -> w304
                  tunnel: [_ _ _ _ _ w507 _ _] -> w303
                  tunnel: w313 -> [_ w414 _ w461 _ w491 _ _]
                  tunnel: [_ w413 _ _ _ _ _ _] -> w300
                  tunnel: [_ _ _ w460 _ _ _ _] -> w297
                  tunnel: [_ _ _ _ _ w490 _ _] -> w294
                  frame #0 {
                    # "AIA, 16 bit, NULL"
                    n109 = To Byte Integer(number=2) -> (8bit integer=w401:i8)
                    n110 = Write to Binary File(file (use dialog)=w412, data="AIA", 5:FALSE ("prepend array or string size? (T)"), 9:T6."little-endian" ("byte order (0:big-endian, network order)")) -> (refnum out=w408:refnum<file>)  [unwired: 2 in, 2 out]
                    n111 = Write to Binary File(file (use dialog)=w408, data=w401, 5:FALSE ("prepend array or string size? (T)"), 9:T6."little-endian" ("byte order (0:big-endian, network order)")) -> (refnum out=w407:refnum<file>)  [unwired: 2 in, 2 out]
                    n112 = To Byte Integer(number=0) -> (8bit integer=w399:i8)
                    n113 = Write to Binary File(file (use dialog)=w407, data=w399, 5:FALSE ("prepend array or string size? (T)"), 9:T6."little-endian" ("byte order (0:big-endian, network order)")) -> ()  [unwired: 2 in, 3 out]
                  }
                  frame #1 {
                    w425 = 0
                    w439 = T6."little-endian" ("byte order (0:big-endian, network order)")
                    n114 = call <userlib>:"CameraGetData.vi"("Data Handle"=w453, "Camera Handle"=w452) -> ("error out"=w455:errorcluster, "Data Handle"=w450:u32)  [unwired: 1 in, 1 out]
                    n115 = To Word Integer(number=3 ("index")) -> (16bit integer=w434:i16)
                    n116 = call <userlib>:"ImageGetArrayI32.vi"("Image Handle"=w450) -> ("Array int 32"=w431:i32[][])  [unwired: 2 in, 2 out]
                    n117 = call <userlib>:"DisplayImage.vi"("error in"=w455, "Image Handle"=w450, "Display Handle"=w454) -> ()  [unwired: 1 in, 2 out]
                    n118 = Array Size(array=w431) -> (size(s)=w432:i32[])
                    n119 = Index Array(array=w432, index=1) -> (element=w436:i32)
                    n120 = Index Array(array=w432, index=0) -> (element=w437:i32)
                    n121 = To Word Integer(number=w431) -> (16bit integer=w430:i16[][])
                    n122 = To Word Integer(number=w437) -> (16bit integer=w438:i16)
                    n123 = To Word Integer(number=w436) -> (16bit integer=w435:i16)
                    n124 = Write to Binary File(file (use dialog)=w446, data=w438, 5:FALSE ("prepend array or string size? (T)"), 9:w439) -> (refnum out=w445:refnum<file>)  [unwired: 2 in, 2 out]
                    n125 = Write to Binary File(file (use dialog)=w445, data=w435, 5:FALSE ("prepend array or string size? (T)"), 9:w439) -> (refnum out=w444:refnum<file>)  [unwired: 2 in, 2 out]
                    n126 = Write to Binary File(file (use dialog)=w444, data=w434, 5:FALSE ("prepend array or string size? (T)"), 9:w439) -> (refnum out=w443:refnum<file>)  [unwired: 2 in, 2 out]
                    n127 = Write to Binary File(file (use dialog)=w443, data=w430, 5:FALSE ("prepend array or string size? (T)"), 9:w439) -> (error out=w449:errorcluster)  [unwired: 2 in, 2 out]
                    n128 = Unbundle(w414) -> (w422:u16[][], "XResAct"=w421:u16, "YResAct"=w420:u16, "BufNrOut"=w419:i16, "BufNrOut"=w418:i16, "ErrorOut"=w417:errorcluster, "hout"=w416:u64, "Bits/pixel"=w415:u16)
                    n129 = call "AddBufferEX.vi"("ph"=w416, "BuffNr"=i16 0, "1stImage"=w425, "LastImage"=w425, "error in (no error)"=w417, "XRes"=w421, "YRes"=w420, "BitPerPixel"=w415) -> ("hout"=w427:u64, "error out"=w426:errorcluster)  [unwired: 5 in, 1 out]
                    n130 = call "WaitForBuffer.vi"("ph"=w427, "sBufNr"=w418, "sBufNr 2"=w419, "timeout"=100, "error in (no error)"=w426) -> ("hout"=w429:u64)  [unwired: 10 in, 4 out]
                    n131 = call "GetImageBuffer2D.vi"("ph"=w429, "BuffIn"=w422, "BuffNr"=i16 0, "xRes"=w421, "yRes"=w420, "Bitresolution"=w415) -> ("BuffOut"=w413:u16[][])  [unwired: 6 in, 3 out]
                  }
                  frame #2 {
                    n132 = Quotient & Remainder(x=w456, y=u32 10) -> (floor(x/y)=w457:u32)  [unwired: 1 out]
                    n133 = Add(x=w457, y=w456) -> (x+y=w459:u32)
                    n134 = Wait (ms)(milliseconds to wait=w459) -> ()  [unwired: 1 out]
                  }
                  frame #3 {
                    w472 = 0
                    n135 = call <userlib>:"CameraGetData.vi"("Data Handle"=w481, "Camera Handle"=w485) -> ("Data Handle"=w480:u32)  [unwired: 1 in, 2 out]
                    n136 = call <userlib>:"DisplayImage.vi"("Image Handle"=w480, "Display Handle"=w482) -> ()  [unwired: 2 in, 2 out]
                    n137 = call <userlib>:"ImageGetArrayI32.vi"("Image Handle"=w480) -> ("Array int 32"=w478:i32[][])  [unwired: 2 in, 2 out]
                    n138 = To Word Integer(number=w478) -> (16bit integer=w477:i16[][])
                    n139 = Write to Binary File(file (use dialog)=w483, data=w477, 5:FALSE ("prepend array or string size? (T)"), 9:T6."little-endian" ("byte order (0:big-endian, network order)")) -> ()  [unwired: 2 in, 3 out]
                    n140 = Unbundle(w461) -> (w469:u16[][], "XResAct"=w468:u16, "YResAct"=w467:u16, "BufNrOut"=w466:i16, "BufNrOut"=w465:i16, "ErrorOut"=w464:errorcluster, "hout"=w463:u64, "Bits/pixel"=w462:u16)
                    n141 = call "AddBufferEX.vi"("ph"=w463, "BuffNr"=i16 0, "1stImage"=w472, "LastImage"=w472, "error in (no error)"=w464, "XRes"=w468, "YRes"=w467, "BitPerPixel"=w462) -> ("hout"=w474:u64, "error out"=w473:errorcluster)  [unwired: 5 in, 1 out]
                    n142 = call "WaitForBuffer.vi"("ph"=w474, "sBufNr"=w465, "sBufNr 2"=w466, "timeout"=100, "error in (no error)"=w473) -> ("hout"=w476:u64)  [unwired: 10 in, 4 out]
                    n143 = call "GetImageBuffer2D.vi"("ph"=w476, "BuffIn"=w469, "BuffNr"=i16 0, "xRes"=w468, "yRes"=w467, "Bitresolution"=w462) -> ("BuffOut"=w460:u16[][])  [unwired: 6 in, 3 out]
                  }
                  frame #4 {
                    n144 = Quotient & Remainder(x=w486, y=u32 10) -> (floor(x/y)=w487:u32)  [unwired: 1 out]
                    n145 = Add(x=w487, y=w486) -> (x+y=w489:u32)
                    n146 = Wait (ms)(milliseconds to wait=w489) -> ()  [unwired: 1 out]
                  }
                  frame #5 {
                    w502 = 0
                    n147 = call <userlib>:"CameraGetData.vi"("Data Handle"=w511, "Camera Handle"=w515) -> ("Data Handle"=w510:u32)  [unwired: 1 in, 2 out]
                    n148 = call <userlib>:"ImageGetArrayI32.vi"("Image Handle"=w510) -> ("Array int 32"=w508:i32[][])  [unwired: 2 in, 2 out]
                    n149 = call <userlib>:"DisplayImage.vi"("Image Handle"=w510, "Display Handle"=w512) -> ()  [unwired: 2 in, 2 out]
                    n150 = To Word Integer(number=w508) -> (16bit integer=w507:i16[][])
                    n151 = Write to Binary File(file (use dialog)=w513, data=w507, 5:FALSE ("prepend array or string size? (T)"), 9:T6."little-endian" ("byte order (0:big-endian, network order)")) -> ()  [unwired: 2 in, 3 out]
                    n152 = Unbundle(w491) -> (w499:u16[][], "XResAct"=w498:u16, "YResAct"=w497:u16, "BufNrOut"=w496:i16, "BufNrOut"=w495:i16, "ErrorOut"=w494:errorcluster, "hout"=w493:u64, "Bits/pixel"=w492:u16)
                    n153 = call "AddBufferEX.vi"("ph"=w493, "BuffNr"=i16 0, "1stImage"=w502, "LastImage"=w502, "error in (no error)"=w494, "XRes"=w498, "YRes"=w497, "BitPerPixel"=w492) -> ("hout"=w504:u64, "error out"=w503:errorcluster)  [unwired: 5 in, 1 out]
                    n154 = call "WaitForBuffer.vi"("ph"=w504, "sBufNr"=w495, "sBufNr 2"=w496, "timeout"=100, "error in (no error)"=w503) -> ("hout"=w506:u64)  [unwired: 10 in, 4 out]
                    n155 = call "GetImageBuffer2D.vi"("ph"=w506, "BuffIn"=w499, "BuffNr"=i16 0, "xRes"=w498, "yRes"=w497, "Bitresolution"=w492) -> ("BuffOut"=w490:u16[][])  [unwired: 6 in, 3 out]
                  }
                  frame #6 {
                    # "Number of replacements is number of lines"
                    n156 = call <vilib>:"System Exec.vi"("command line"="php C:\\Users\\BECV\\Documents\\DAS\\dbquery.php") -> ("standard output"=w524:string)  [unwired: 7 in, 3 out]
                    n157 = Search and Replace String(replace all?=TRUE ("replace all? (F)"), input string=w524, search string="(") -> (result string=w522:string)  [unwired: 5 in, 3 out]
                    n158 = Search and Replace String(replace all?=TRUE ("replace all? (F)"), input string=w522, search string=")") -> (result string=w518:string, number of replacements=w516:i32)  [unwired: 5 in, 2 out]
                    "Database Output" <- w518
                    n159 = for {
                      N: w516 -> [_]
                      tunnel: w518 -> [w545]
                      tunnel: w517 -> [w541]
                      i -> [w546]
                      w533 = T6."little-endian" ("byte order (0:big-endian, network order)")
                      n160 = Pick Line(multi-line string=w545, line index=w546) -> (output string=w544:string)  [unwired: 1 in]
                      n161 = Match Pattern(string=w544, regular expression="\\s") -> (before substring=w536:string, after substring=w542:string)  [unwired: 1 in, 2 out]
                      n162 = Fract/Exp String To Number(string=w542) -> (number=w530:dbl)  [unwired: 3 in, 1 out]
                      n163 = Concatenate Strings(w536) -> (w535:string)
                      n164 = To Byte Integer(number=0) -> (8bit integer=w527:i8)
                      n165 = To Double Precision Float(number=w530) -> (double precision float=w528:dbl)
                      n166 = Write to Binary File(file (use dialog)=w541, data=w535, 5:FALSE ("prepend array or string size? (T)"), 9:w533) -> (refnum out=w537:refnum<file>, error out=w538:errorcluster)  [unwired: 2 in, 1 out]
                      n167 = Write to Binary File(file (use dialog)=w537, data=w527, error in=w538, 5:FALSE ("prepend array or string size? (T)"), 9:T6."little-endian" ("byte order (0:big-endian, network order)")) -> (refnum out=w531:refnum<file>, error out=w534:errorcluster)  [unwired: 1 in, 1 out]
                      n168 = Write to Binary File(file (use dialog)=w531, data=w528, error in=w534, 5:FALSE ("prepend array or string size? (T)"), 9:w533) -> ()  [unwired: 1 in, 3 out]
                    }
                  }
                  frame #7 {
                    n169 = Close File(refnum=w547) -> ()  [unwired: 1 in, 2 out]
                  }
                }
                n170 = for {
                  N -> [w355]
                  shift-right: [w356] -> w299
                  shift-left: w300 -> [w358]
                  tunnel: w300 -> [w357] mode=indexing
                  i -> [w351]
                  n171 = Subtract(x=w355, y=1) -> (x-y=w353:i32)
                  n172 = Subtract(x=w353, y=w351) -> (x-y=w352:i32)
                  n173 = Replace Array Subset(array=w358, new element=w357, index (row)=w352) -> (w356:u16[][])  [unwired: 1 in]
                }
                n174 = Transpose 2D Array(2D array=w299) -> (transposed array=→"PF Atoms":u16[][])
                n175 = for {
                  N -> [w379]
                  shift-right: [w380] -> w308
                  shift-left: w309 -> [w382]
                  tunnel: w309 -> [w381] mode=indexing
                  i -> [w375]
                  n176 = Subtract(x=w379, y=1) -> (x-y=w377:i32)
                  n177 = Subtract(x=w377, y=w375) -> (x-y=w376:i32)
                  n178 = Replace Array Subset(array=w382, new element=w381, index (row)=w376) -> (w380:i16[][])  [unwired: 1 in]
                }
                n179 = for {
                  N -> [w347]
                  shift-right: [w348] -> w296
                  shift-left: w297 -> [w350]
                  tunnel: w297 -> [w349] mode=indexing
                  i -> [w343]
                  n180 = Subtract(x=w347, y=1) -> (x-y=w345:i32)
                  n181 = Subtract(x=w345, y=w343) -> (x-y=w344:i32)
                  n182 = Replace Array Subset(array=w350, new element=w349, index (row)=w344) -> (w348:u16[][])  [unwired: 1 in]
                }
                n183 = Transpose 2D Array(2D array=w308) -> (transposed array=→"Atoms":i16[][])
                n184 = Transpose 2D Array(2D array=w296) -> (transposed array=→"PF No Atoms":u16[][])
                n185 = Subtract(x=w309, y=w303) -> (x-y=w321:i16[][])
                n186 = for {
                  N -> [w339]
                  shift-right: [w340] -> w293
                  shift-left: w294 -> [w342]
                  tunnel: w294 -> [w341] mode=indexing
                  i -> [w335]
                  n187 = Subtract(x=w339, y=1) -> (x-y=w337:i32)
                  n188 = Subtract(x=w337, y=w335) -> (x-y=w336:i32)
                  n189 = Replace Array Subset(array=w342, new element=w341, index (row)=w336) -> (w340:u16[][])  [unwired: 1 in]
                }
                n190 = for {
                  N -> [w371]
                  shift-right: [w372] -> w306
                  shift-left: w304 -> [w374]
                  tunnel: w304 -> [w373] mode=indexing
                  i -> [w367]
                  n191 = Subtract(x=w371, y=1) -> (x-y=w369:i32)
                  n192 = Subtract(x=w369, y=w367) -> (x-y=w368:i32)
                  n193 = Replace Array Subset(array=w374, new element=w373, index (row)=w368) -> (w372:i16[][])  [unwired: 1 in]
                }
                n194 = Subtract(x=w304, y=w303) -> (x-y=w320:i16[][])
                n195 = Transpose 2D Array(2D array=w306) -> (transposed array=→"No Atoms":i16[][])
                n196 = Subtract(x=w297, y=w294) -> (x-y=w288:u16[][])
                n197 = Multiply(x=w288, y="PF Scale") -> (x*y=w287:dbl[][])
                n198 = Multiply(x=w320, y="Scaling") -> (x*y=w319:dbl[][])
                n199 = Subtract(x=w300, y=w294) -> (x-y=w286:u16[][])
                n200 = Divide(x=w286, y=w287) -> (x/y=w311:dbl[][])
                n201 = Divide(x=w321, y=w319) -> (x/y=w317:dbl[][])
                n202 = for {
                  N -> [w363]
                  shift-right: [w364] -> w302
                  shift-left: w303 -> [w366]
                  tunnel: w303 -> [w365] mode=indexing
                  i -> [w359]
                  n203 = Subtract(x=w363, y=1) -> (x-y=w361:i32)
                  n204 = Subtract(x=w361, y=w359) -> (x-y=w360:i32)
                  n205 = Replace Array Subset(array=w366, new element=w365, index (row)=w360) -> (w364:i16[][])  [unwired: 1 in]
                }
                n206 = for {
                  N -> [w388]
                  shift-right: [w389] -> w312
                  shift-left: w311 -> [w390]
                  tunnel: w311 -> [w383] mode=indexing
                  i -> [w384]
                  n207 = Subtract(x=w388, y=1) -> (x-y=w386:i32)
                  n208 = Subtract(x=w386, y=w384) -> (x-y=w385:i32)
                  n209 = Replace Array Subset(array=w390, new element=w383, index (row)=w385) -> (w389:dbl[][])  [unwired: 1 in]
                }
                n210 = Transpose 2D Array(2D array=w293) -> (transposed array=→"PF Dark":u16[][])
                n211 = Array Size(array=w317) -> ()  [unwired: 1 out]
                n212 = for {
                  N -> [w395]
                  shift-right: [w396] -> w318
                  shift-left: w317 -> [w398]
                  tunnel: w317 -> [w397] mode=indexing
                  i -> [w391]
                  n213 = Subtract(x=w395, y=1) -> (x-y=w393:i32)
                  n214 = Subtract(x=w393, y=w391) -> (x-y=w392:i32)
                  n215 = Replace Array Subset(array=w398, new element=w397, index (row)=w392) -> (w396:dbl[][])  [unwired: 1 in]
                }
                n216 = Transpose 2D Array(2D array=w302) -> (transposed array=→"Dark Field":i16[][])
                n217 = Transpose 2D Array(2D array=w312) -> (transposed array=→"Intensity Graph":dbl[][])
                n218 = Transpose 2D Array(2D array=w318) -> (transposed array=→"Normalized Image":dbl[][])
              }
            }
            n219 = Split Signals(w271) -> (w270:dynamicdata)  [unwired: 3 in, 2 out]
            n220 = Multiply(x=w270, y=1.021) -> (x*y=w268:dynamicdata)
            n221 = Add(x=-0.5356, y=w268) -> (x+y=→"Top of Chamber Monitor":dynamicdata)
            n222 = Not(x="?") -> (.not. x?=w263:bool)
            n223 = And(x=w265, y=w263) -> (x .and. y?=w264:bool)
          }
        }
      }
      n224 = Wait (ms)(milliseconds to wait=u32 5) -> ()  [unwired: 1 out]
    }
    frame #3 {
      w554 = u16 0 items=["Stop", "Run"] ("RecordingState")
      # "CoolSnapHQ"
      # "Stop recording"
      # "Step 3:\nClose the handles."
      n225 = call "CancelImages.vi"("ph"=w553) -> ("error out"=w556:errorcluster, "hout"=w555:u64)  [unwired: 2 in, 1 out]
      n226 = call "SetRecordingState.vi"("ErrorIn"=w556, "RecordingState"=w554, "ph"=w555) -> ("ErrorOut"=w548:errorcluster, "hout"=w549:u64)  [unwired: 2 in, 1 out]
      n227 = call "ExSubCloseExperimentCoolSnap.vi"("Handles In"=w557) -> ()  [unwired: 1 in, 1 out]
      n228 = call "Cleanup.vi"("error in (no error)"=w548, "ph"=w549) -> ("error out"=w551:errorcluster, "hout"=w550:u64)  [unwired: 8 in]
      n229 = call "CloseCamera.vi"("ErrorIn"=w551, "Handle in"=w550) -> ("ErrorOut"=w552:errorcluster)  [unwired: 1 in, 2 out]
      n230 = call <vilib>:"Simple Error Handler.vi"("error in (no error)"=w552) -> ()  [unwired: 4 in, 5 out]
    }
  }
